vi "ProdaNG.Units.FindById.vi"(0 "units":T1[](array[typedef]), 1 "unit id":i32, 2 "add brackets (F)":bool) -> (3 "unit str":string)   [LabVIEW 2016]
uses:
  Controls/ProdaNG.UnitSimple.ctl
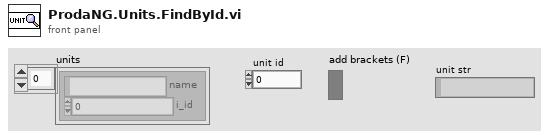
[diagram p1: front panel]
types:
  T1 = typedef "ProdaNG.UnitSimple.ctl" = cluster{"name":string, "i_id":i32}
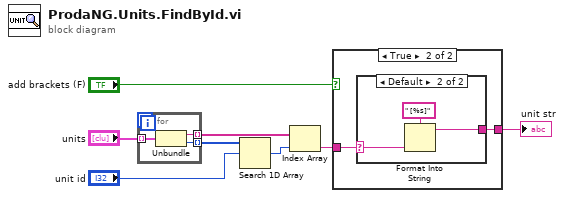
[diagram p0: block diagram]
diagram:
  n1 = for {
    tunnel: [w11] -> w5 mode=indexing
    tunnel: [w10] -> w6 mode=indexing
    tunnel: "units" -> [w9] mode=indexing
    n2 = Unbundle(w9) -> ("name"=w11:string, "i_id"=w10:i32)
  }
  n3 = Search 1D Array(1D array=w6, element="unit id") -> (index of element=w8:i32)  [unwired: 1 in]
  n4 = Index Array(array=w5, index=w8) -> (element=w3:string)
  n5 = case shown="True" "add brackets (F)" {
    tunnel: w3 -> [w12 w14]
    tunnel: [w12 w13] -> w2
    frame False {
    }
    frame True {
      n6 = case shown="Default" w14 {
        selector: w14 -> [_ w17]
        tunnel: [_ w15] -> w13
        frame "", "-", "bool", "digit" {
        }
        frame Default {
          n7 = Format Into String(format string=" [%s]", w17) -> (resulting string=w15:string)  [unwired: 2 in, 1 out]
        }
      }
    }
  }
  "unit str" <- w2
